vi "writeVelocityFirgelli.vi"(8 "error in (no error)":errorcluster, 10 "Velocity":dbl(slide) scale=0.0..100.0, 11 "handleIn":u32 format="%x") -> (0 "error out":errorcluster, 1 "regSetting":u16, 2 "pDataOut":u8[](array[numeric]), 3 "handleOut":u32 format="%x")   [LabVIEW 2016]
doc: "0x0A SET_MAX_PWM_VALUE\nThis is the value that is manually controlled by the speed potentiometer. This is the speed that the actuator runs at when outside the PWM_THRESHOLD. Setting this to 1023 will allow the actuator to achieve full speed. The actuator may exceed this value while attempting to overcome a stall condition.\n\nWritten by: Complete Automated Solutions\nwww.CompleteAutomatedSolutions.com"
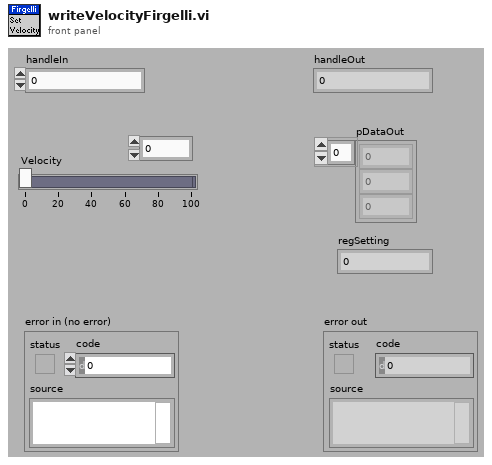
[diagram p1: front panel]
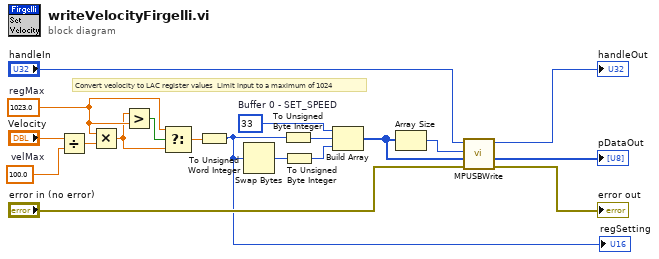
[diagram p0: block diagram]
diagram:
  w8 = 100.0  # velMax
  w2 = 1023.0  # regMax
  w16 = u8 33  # Buffer 0 - SET_SPEED
  # "Convert veolocity to LAC register values  Limit input to a maximum of 1024"
  n1 = Divide(x="Velocity", y=w8) -> (x/y=w7:dbl)
  n2 = Multiply(x=w2, y=w7) -> (x*y=w1:dbl)
  n3 = Greater?(x=w1, y=w2) -> (0:w4:bool)
  n4 = Select(t=w2, s=w4, f=w1) -> (s? t:f=w3:dbl)
  n5 = To Unsigned Word Integer(number=w3) -> (unsigned 16bit integer=w6:u16)
  "regSetting" <- w6
  n6 = Swap Bytes(anything=w6) -> (byte swapped=w19:u16)
  n7 = To Unsigned Byte Integer(number=w6) -> (unsigned 8bit integer=w17:u8)
  n8 = To Unsigned Byte Integer(number=w19) -> (unsigned 8bit integer=w18:u8)
  n9 = Build Array(w16, w17, w18) -> (w14:u8[])
  n10 = Array Size(array=w14) -> (size(s)=w15:i32)
  n11 = call "MPUSBWrite.vi"("error in (no error)"="error in (no error)", "pDataIn"=w14, "dwLen"=w15, "handleIn"="handleIn") -> ("error out"=→"error out":errorcluster, "pDataOut"=→"pDataOut":u8[], "handleOut"=→"handleOut":u32)  [unwired: 2 in, 3 out]
